vi "Compile.vi"(8 "INO":path, 11 "CLI":path) -> (2 "concatenated string":string)   [LabVIEW 2025]
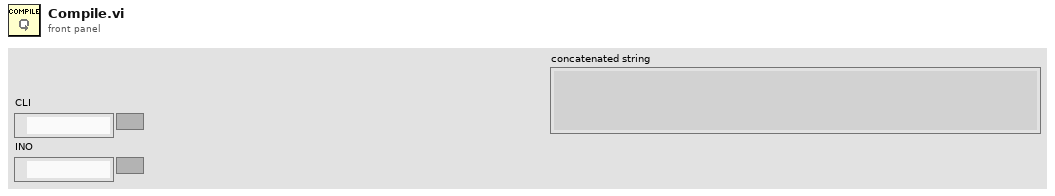
[diagram p1: front panel]
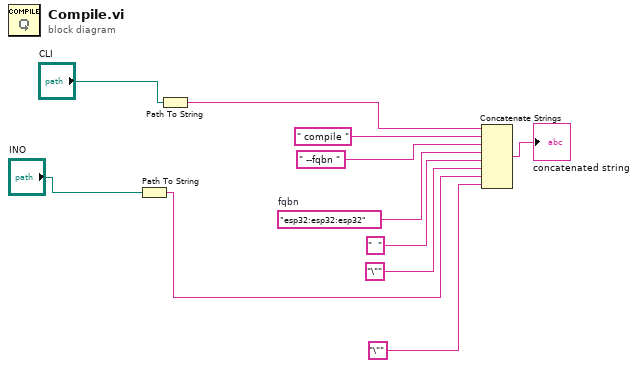
[diagram p0: block diagram]
diagram:
  w7 = "esp32:esp32:esp32"  # fqbn
  n1 = Path To String(path="INO") -> (string=w4:string)
  n2 = Path To String(path="CLI") -> (string=w10:string)
  n3 = Concatenate Strings(w10, " compile " ("string"), " --fqbn " ("string"), w7, "  " ("string"), "\"" ("string"), w4, "\"" ("string")) -> (→"concatenated string":string)
